vi "Drive Stright.vi"(8 "Dead Zone":dbl, 9 "Force Straight":bool, 10 "Left Joystick":dbl, 11 "Right Joystick":dbl) -> (2 "Left Drive Output":dbl, 3 "Right Drive Output":dbl)   [LabVIEW 2016]
doc: "This VI will help the driver get the joystick values to be equal. If the input values are within the deadzone of eachother they will be averaged and sent to the output. The force stright button will ignore the deadzone when pressed.\n\nCreated by Team 4130 for use in the 2016-2017 FRC season"
uses:
  <vilib>/Analysis/baseanly.llb/Mean (DBL).vi
  <vilib>/Analysis/NI_AALBase.lvlib
panel:
  # "If the Values of the input are within Deadline of eachother then Both motors recieve the same value"
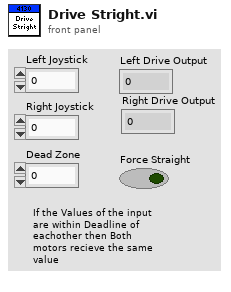
[diagram p1: front panel]
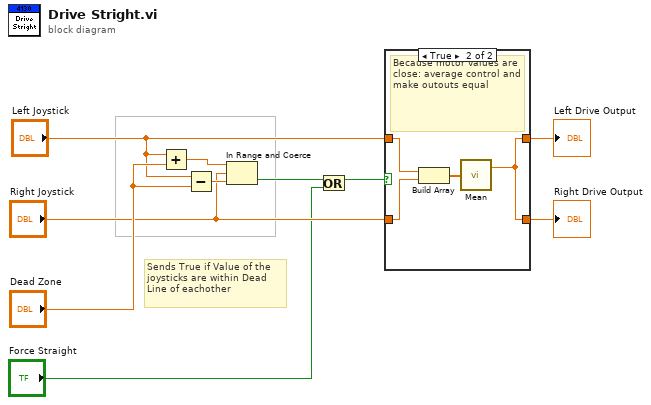
[diagram p0: block diagram]
diagram:
  # "Sends True if Value of the joysticks are within Dead Line of eachother"
  n1 = Add(x="Left Joystick", y="Dead Zone") -> (x+y=w10:dbl)
  n2 = Subtract(x="Left Joystick", y="Dead Zone") -> (x-y=w8:dbl)
  n3 = In Range and Coerce(upper limit=w10, x="Right Joystick", lower limit=w8) -> (In Range?=w3:bool)  [unwired: 1 out]
  n4 = Or(x=w3, y="Force Straight") -> (x .or. y?=w2:bool)
  n5 = case shown="True" w2 {
    tunnel: [w12 w13] -> w7
    tunnel: "Left Joystick" -> [w12 w16]
    tunnel: [w11 w13] -> w5
    tunnel: "Right Joystick" -> [w11 w15]
    frame False {
      # "The motor output values recived by this VI are not close in value: send the Raw input Out"
    }
    frame True {
      # "Because motor values are close: average control and make outouts equal"
      n6 = Build Array(w16, w15) -> (w14:dbl[])
      n7 = call-poly <vilib>:"Mean.vi"("X"=w14) -> ("mean"=w13:dbl)  [unwired: 1 out]
    }
  }
  "Left Drive Output" <- w7
  "Right Drive Output" <- w5
